vi "User Event Data.vi"(7 "Data Functions":T2, 8 "error in (no error)":errorcluster) -> (0 "error out":errorcluster, 3 "User Event Data":T1)   [LabVIEW 2016, in "System.lvlib"]
uses:
  System.lvlib
  Controls/Control_Data Functions.ctl
  Controls/Control_User Event.ctl
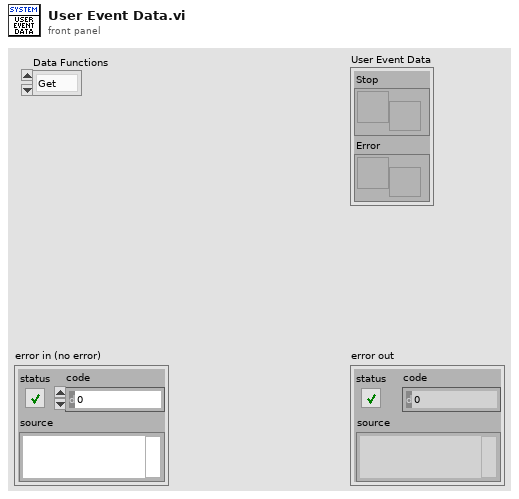
[diagram p1: front panel]
types:
  T1 = typedef "System.lvlib/Control_User Event.ctl" = cluster{"Stop":refnum<user-event>, "Error":refnum<user-event>}
  T2 = typedef "System.lvlib/Control_Data Functions.ctl" = enum16{"Get", "Set", "Release"}
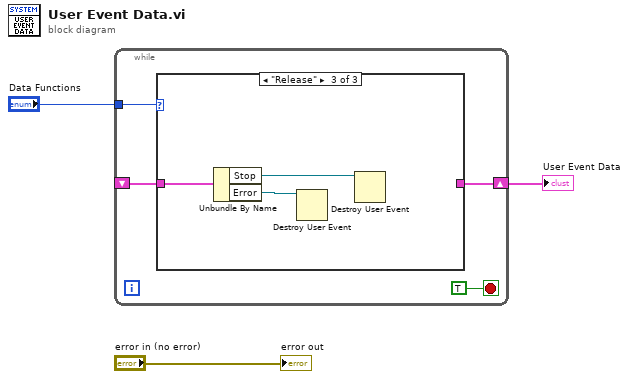
[diagram p0: block diagram]
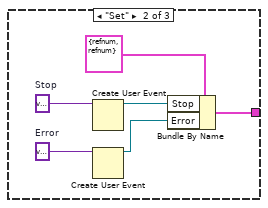
[diagram p3: hidden frame]
diagram:
  n1 = while {
    tunnel: "Data Functions" -> [w6]
    shift-right: [w4] -> w1
    shift-left: _ -> [w5]
    stop <- TRUE stop-if-true
    n2 = case shown="\"Release\"" w6 {
      tunnel: w5 -> [w8 _ w17]
      tunnel: [w8 w11 _] -> w4
      frame "Get", Default {
      }
      frame "Set" {
        w9 = variant  # Error
        w10 = variant  # Stop
        n3 = Create User Event(user event datatype=w10) -> (user event=w13:refnum<user-event>)  [unwired: 1 in, 1 out]
        n4 = Create User Event(user event datatype=w9) -> (user event=w14:refnum<user-event>)  [unwired: 1 in, 1 out]
        n5 = Bundle By Name(cluster=T1 {"Stop"=refnum, "Error"=refnum} ("User Event"), "Stop"=w13, "Error"=w14) -> (w11:T1)
      }
      frame "Release" {
        n6 = Unbundle By Name(w17) -> ("Stop"=w15:refnum<user-event>, "Error"=w16:refnum<user-event>)
        n7 = Destroy User Event(user event=w16) -> ()  [unwired: 1 in, 1 out]
        n8 = Destroy User Event(user event=w15) -> ()  [unwired: 1 in, 1 out]
      }
    }
  }
  "User Event Data" <- w1
  "error out" <- "error in (no error)"
